vi "4 - Potências de 2.vi"() -> ()   [LabVIEW 2020]
panel:
  in  "Boolean":bool
  out "Numeric 5":dbl
  out "Numeric 4":dbl
  out "Numeric 3":dbl
  out "Numeric 2":dbl
  out "Numeric":dbl
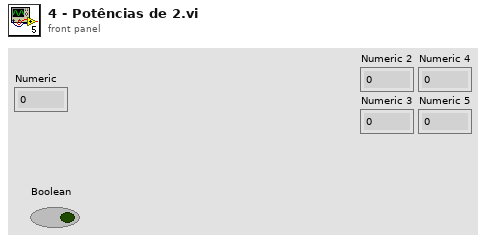
[diagram p1: front panel]
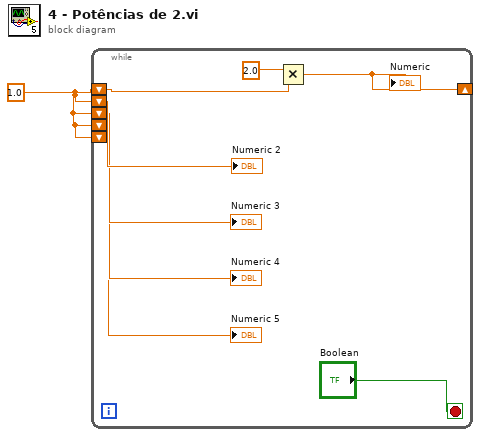
[diagram p0: block diagram]
diagram:
  w1 = 1.0
  n1 = while {
    shift-right: [w7] -> _
    shift-left: w1 -> [w8]
    shift-left: w1 -> [w6]
    shift-left: w1 -> [w5]
    shift-left: w1 -> [w4]
    shift-left: w1 -> [w3]
    stop <- "Boolean" stop-if-true
    n2 = Multiply(x=2.0, y=w8) -> (x*y=w7:dbl)
    "Numeric" <- w7
    "Numeric 2" <- w6
    "Numeric 3" <- w5
    "Numeric 4" <- w4
    "Numeric 5" <- w3
  }
